vi "Get Position Params.vi"(8 "error in (no error)":errorcluster, 11 "VacuumLine Configuration in":refnum<class "VacuumLine Configuration.lvclass">) -> (0 "error out":errorcluster, 2 "Position Params":T1 {"max( |Motor Pos - LRF Distance| )" min=0.0}, 3 "VacuumLine Configuration out":refnum<class "VacuumLine Configuration.lvclass">)   [LabVIEW 2016, in "Hardware.lvlib" / "VacuumLine.lvlib" / "VacuumLine Configuration.lvclass"]
uses:
  <userlib>/Common Components/Hardware/Abstract System/VacuumLine/VacuumLine Config/VacuumLine Configuration.lvclass
  <userlib>/Common Components/Hardware/Abstract System/VacuumLine/VacuumLine/VacuumLine Params.ctl
  <userlib>/Common Components/Hardware/Abstract System/VacuumLine/VacuumLine/Valve Complex.ctl
  <userlib>/Common Components/Hardware/Abstract System/VacuumLine/VacuumLine/Logic Cluster.ctl
  <userlib>/Common Components/Hardware/Abstract System/VacuumLine/VacuumLine Config/VacuumLine Configuration.lvclass/VacuumLine Configuration.ctl
  <userlib>/Common Components/Hardware/Abstract System/VacuumLine/VacuumLine/VacuumLine.lvclass/VacuumLine.ctl
  <userlib>/Common Components/Hardware/Abstract System/VacuumLine/VacuumLine/VacuumLine.lvclass
panel:
  # "Pin#"
  # "Location"
  # "Tolerance"
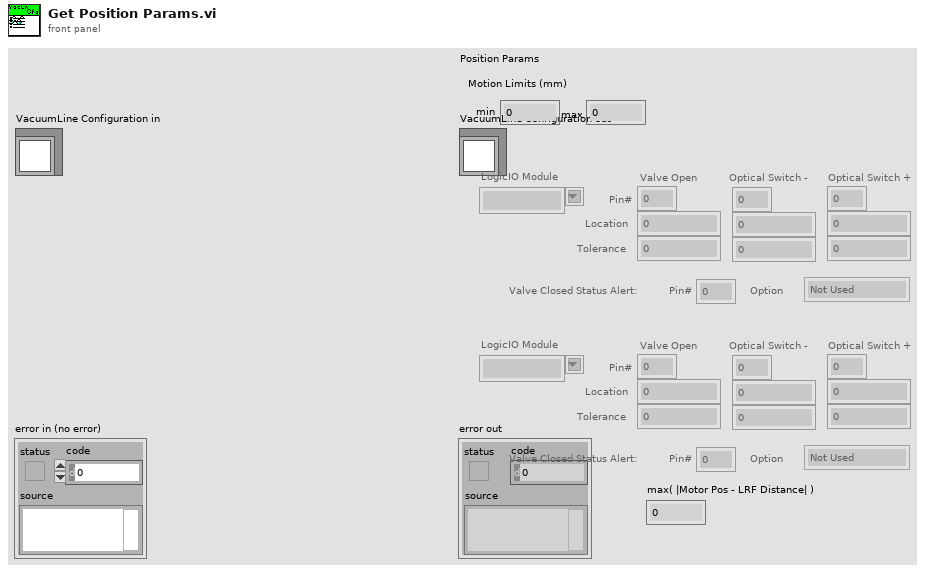
[diagram p1: front panel]
types:
  T1 = typedef "Hardware.lvlib/VacuumLine.lvlib/VacuumLine.lvclass/VacuumLine Params.ctl" = cluster{"Motion Limits":cluster{"min":dbl, "max":dbl}, "Valve Complexes":T2[], "max( |Motor Pos - LRF Distance| )":dbl}
  T2 = typedef "Hardware.lvlib/VacuumLine.lvlib/VacuumLine.lvclass/Valve Complex.ctl" = cluster{"LogicIO Module":string, "Valve Open":T3, "Optical Switch -":T3, "Optical Switch +":T3, "Valve Closed Status Alert":cluster{"Pin#":u8, "Option":enum16{"Not Used", "Normally Closed"}}}
  T3 = typedef "Hardware.lvlib/VacuumLine.lvlib/VacuumLine.lvclass/Logic Cluster.ctl" = cluster{"Pin#":u8, "Location":dbl, "Tolerance":dbl}
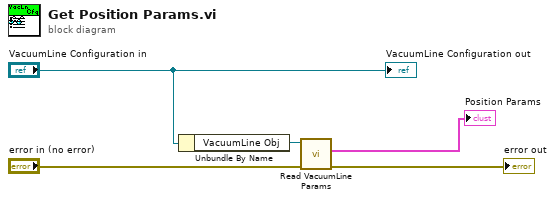
[diagram p0: block diagram]
diagram:
  n1 = Unbundle By Name("VacuumLine Configuration in") -> ("VacuumLine Obj"=w1:refnum<class "VacuumLine.lvclass">)
  n2 = call <userlib>:"Read VacuumLine Params.vi"("error in (no error)"="error in (no error)", "VacuumLine in"=w1) -> ("error out"=→"error out":errorcluster, "Position Params"=→"Position Params":T1)  [unwired: 7 in, 1 out]
  "VacuumLine Configuration out" <- "VacuumLine Configuration in"
